vi "Liaison Série - 2 cam 1P.vi"(9 "timeout (ms)":u32=500, 11 "Port USB en réception":refnum<visa-resource-name>="ASRL1::INSTR") -> (2 "Indications pokaenmon D":T1, 3 "Indications pokaenmon G":T1, 4 "Nom VISA en sortie":refnum<visa-resource-name>)   [LabVIEW 2013]
uses:
  <vilib>/Instr/_visa.llb/VISA Configure Serial Port (Instr).vi
panel:
  out "error out":errorcluster caption="sortie d'erreur"
  out "Sortie lue":string
  # "Réception de données-XBee"
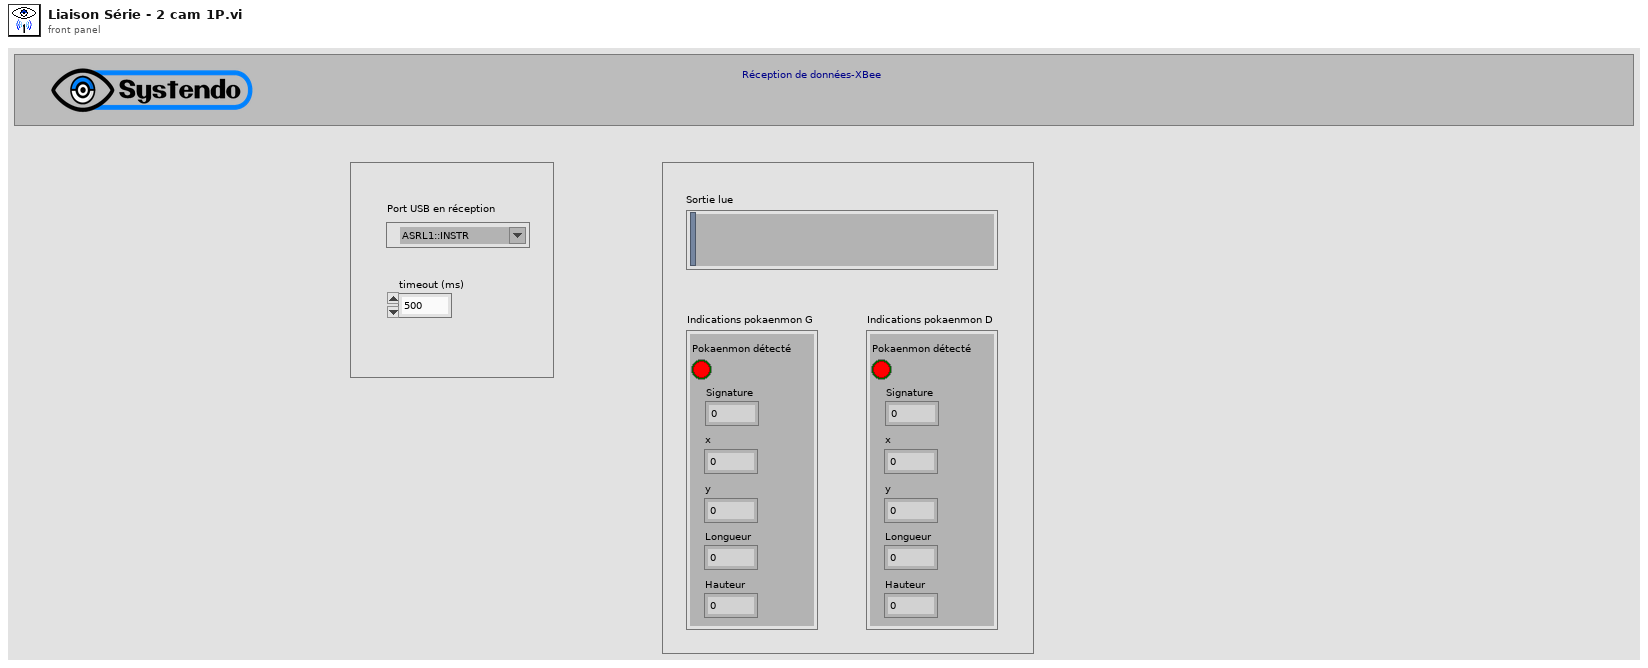
[diagram p1: front panel]
types:
  T1 = cluster{"Pokaenmon détecté":bool, "Signature":u32, "x":dbl, "y ":dbl, "Longueur":dbl, "Hauteur":dbl}
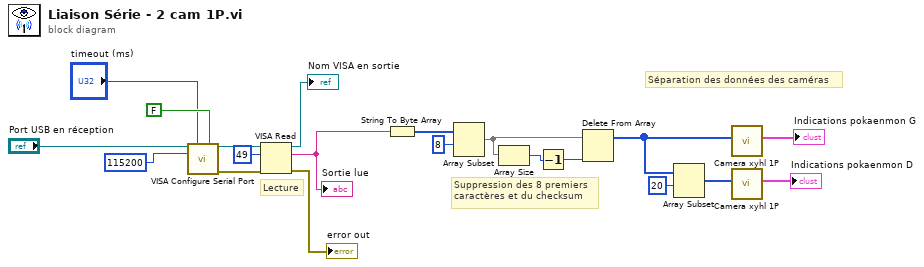
[diagram p0: block diagram]
diagram:
  # "Séparation des données des caméras"
  # "Suppression des 8 premiers\ncaractères et du checksum"
  # "Lecture"
  n1 = call-poly "VISA Configure Serial Port"("VISA resource name"="Port USB en réception", "timeout (10sec)"="timeout (ms)", "Enable Termination\nChar (T)"=FALSE ("Enable Termination\nChar (T)"), "baud rate (9600)"=u32 115200 ("Baud Rate (115200)")) -> ("VISA resource name out"=w13:refnum<visa-resource-name>, "error out"=w11:errorcluster)  [unwired: 10 in]
  n2 = VISA Read(VISA resource name=w13, byte count=u32 49 ("nombre d'octets"), error in (no error)=w11) -> (VISA resource name out=→"Nom VISA en sortie":refnum<visa-resource-name>, read buffer=w20:string, error out=→"error out":errorcluster)  [unwired: 1 out]
  "Sortie lue" <- w20
  n3 = String To Byte Array(string=w20) -> (unsigned byte array=w19:u8[])
  n4 = Array Subset(array=w19, index=8 ("offset (0)")) -> (w9:u8[])  [unwired: 1 in]
  n5 = Array Size(array=w9) -> (size(s)=w2:i32)
  n6 = Decrement(x=w2) -> (x-1=w1:i32)
  n7 = Delete From Array(array=w9, index=w1) -> (array with subset deleted=w3:u8[])  [unwired: 1 in, 1 out]
  n8 = Array Subset(array=w3, index=20 ("indice")) -> (w6:u8[])  [unwired: 1 in]
  n9 = call "Camera xyhl 1P.vi"("tableau"=w3) -> ("Indications pokaenmon"=→"Indications pokaenmon G":T1)  [unwired: 10 in]
  n10 = call "Camera xyhl 1P.vi"("tableau"=w6) -> ("Indications pokaenmon"=→"Indications pokaenmon D":T1)  [unwired: 10 in]
